vi "FGGA TCP Packet_v3.vi"(7 "TCP Packet In":string, 12 "Data Array":string[](array[string])) -> (8 "TCP Binary Packet":string)   [LabVIEW 2014]
panel:
  out "array":string[](array[string])
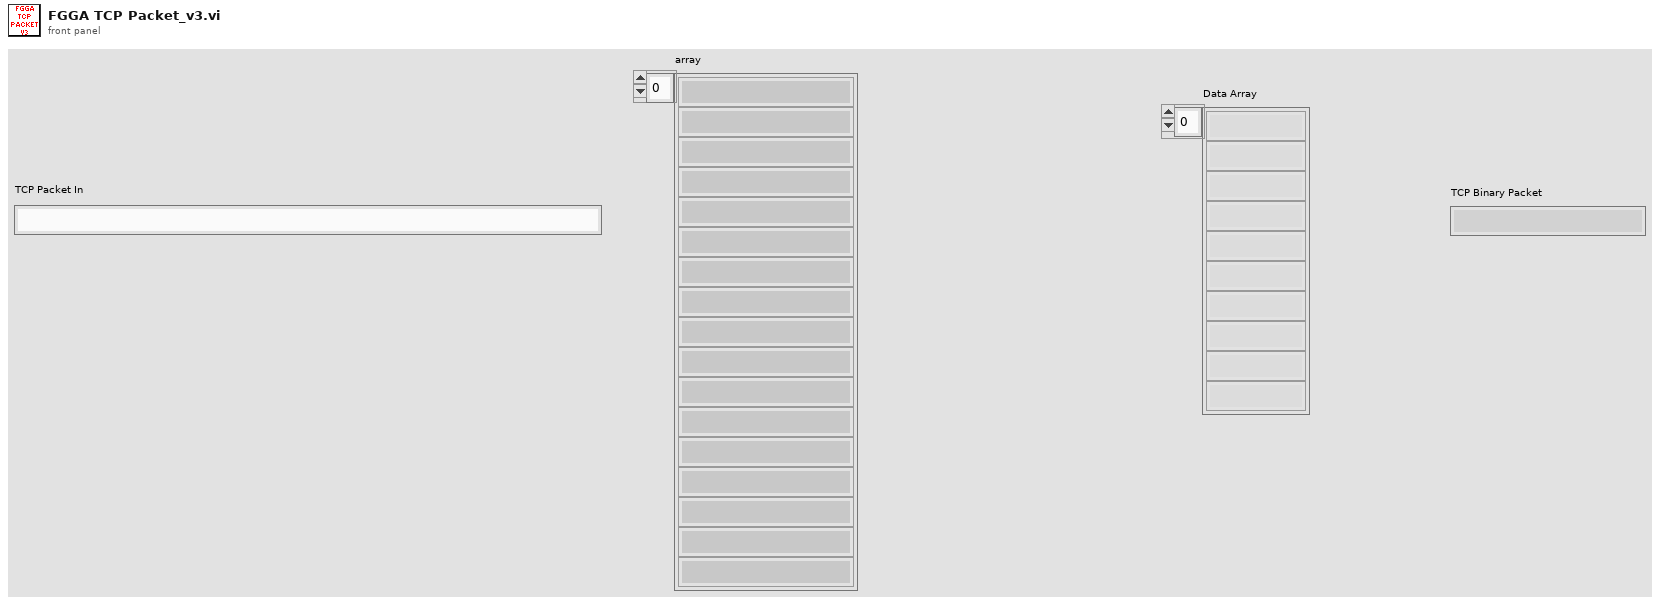
[diagram p1: front panel]
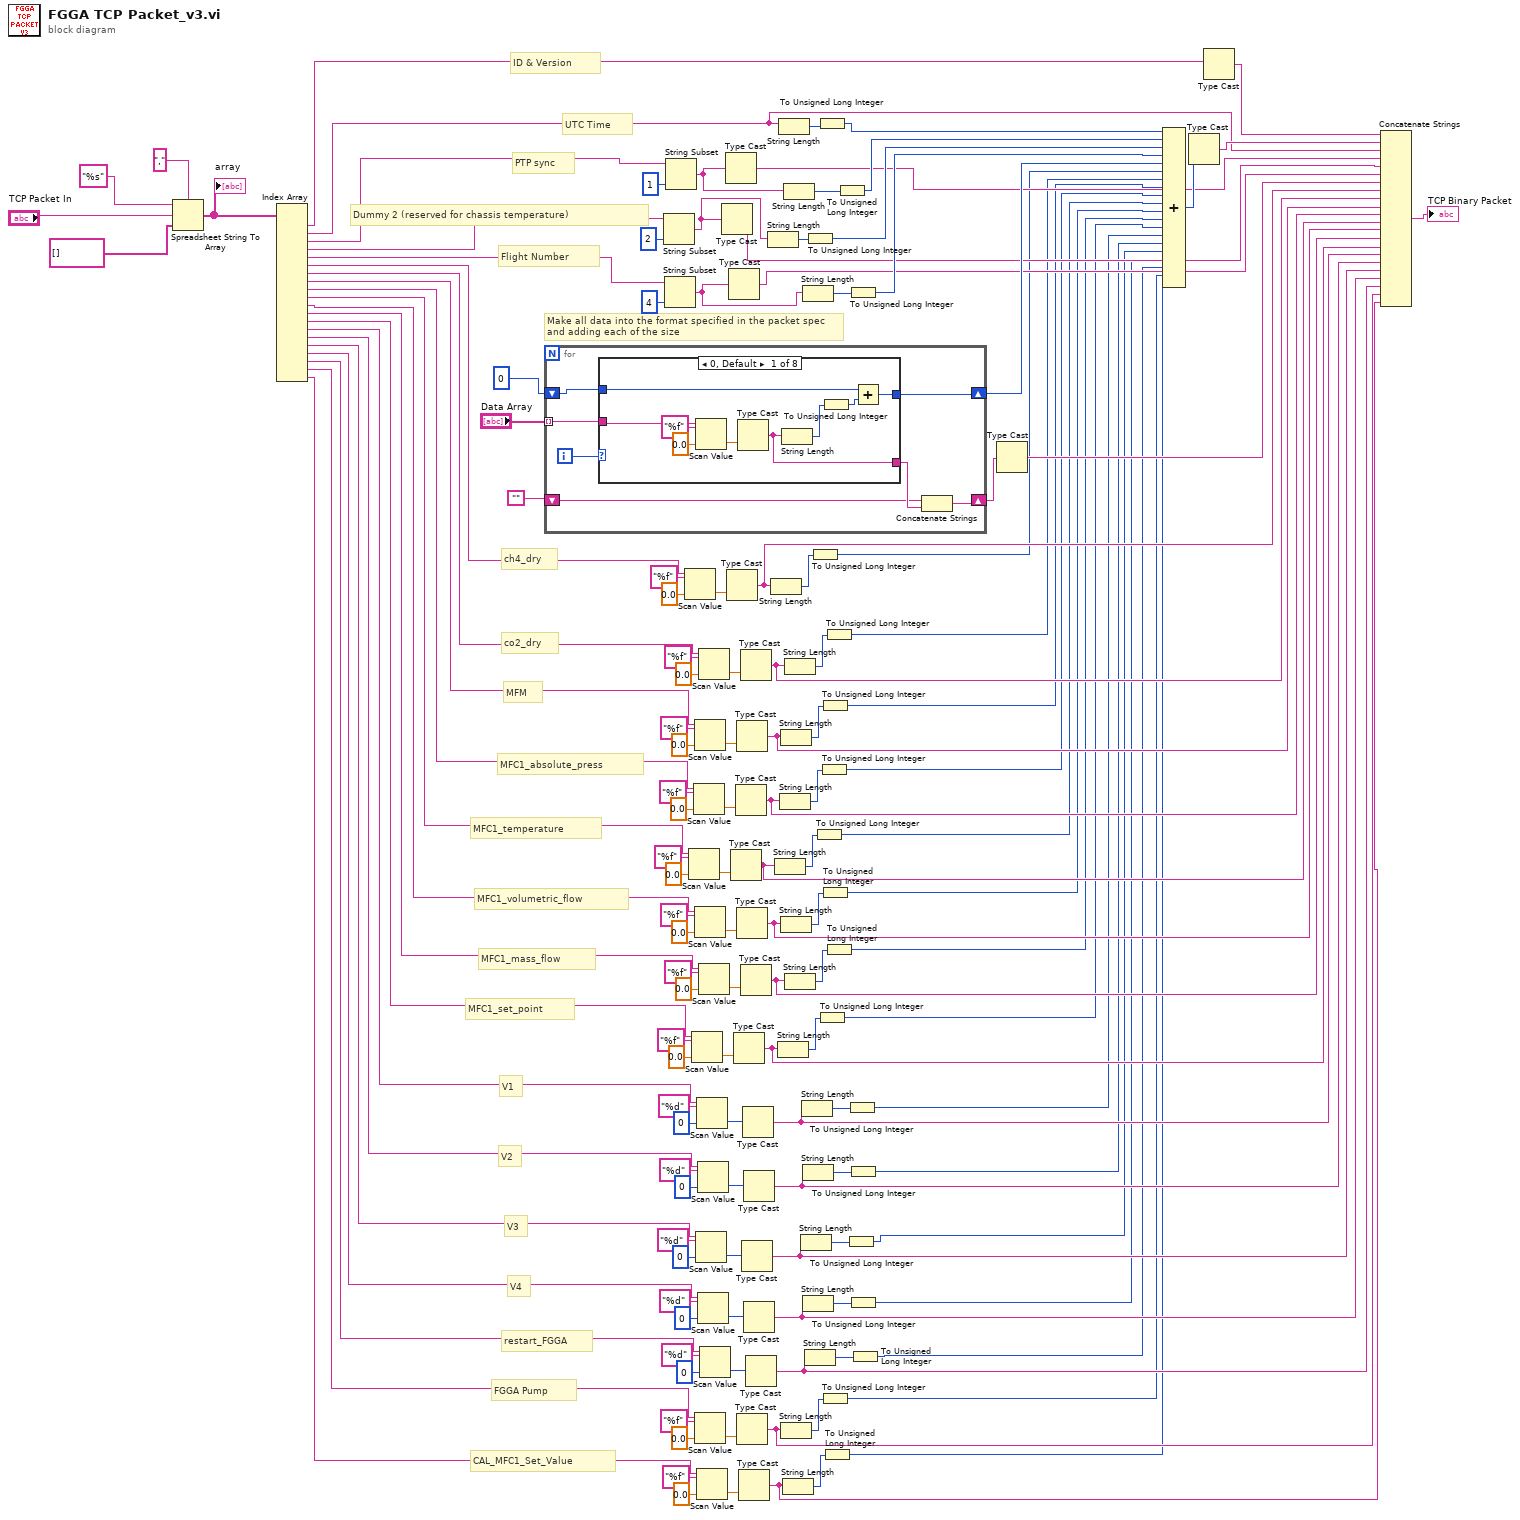
[diagram p0: block diagram]
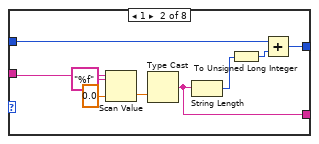
[diagram p2: hidden frame]
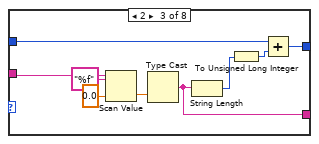
[diagram p3: hidden frame]
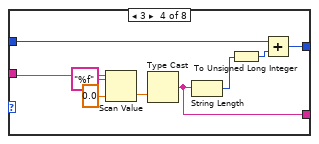
[diagram p4: hidden frame]
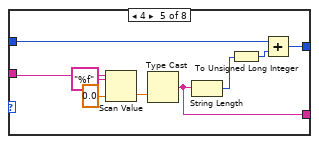
[diagram p5: hidden frame]
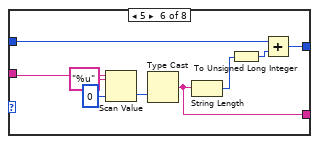
[diagram p6: hidden frame]
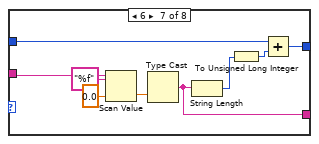
[diagram p7: hidden frame]
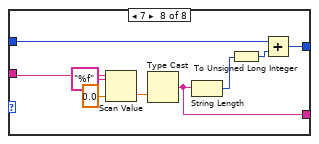
[diagram p8: hidden frame]
diagram:
  # "PTP sync"
  # "CAL_MFC1_Set_Value"
  # "FGGA Pump"
  # "restart_FGGA"
  # "V4"
  # "V3"
  # "V2"
  # "V1"
  # "MFC1_set_point"
  # "MFC1_mass_flow"
  # "MFC1_volumetric_flow"
  # "MFC1_temperature"
  # "MFC1_absolute_press"
  # "MFM"
  # "co2_dry"
  # "ch4_dry"
  # "Flight Number"
  # "Dummy 2 (reserved for chassis temperature)"
  # "UTC Time"
  # "ID & Version"
  # "Make all data into the format specified in the packet spec\nand adding each of the size"
  n1 = Spreadsheet String To Array(delimiter (Tab)=",", format string="%s", spreadsheet string="TCP Packet In", array type (2D Dbl)=string[] []) -> (array=w99:string[])
  "array" <- w99
  n2 = Index Array(array=w99) -> (element #1=w98:string, element #2=w97:string, element #3=w96:string, element #4=w95:string, element #5=w94:string, element #6=w93:string, element #7=w92:string, element #8=w67:string, element #9=w64:string, element #10=w61:string, element #11=w58:string, element #12=w55:string, element #13=w52:string, element #14=w45:string, element #15=w38:string, element #16=w15:string, element #17=w12:string, element #18=w9:string, element #19=w6:string, element #20=w3:string)  [unwired: 20 in]
  n3 = for {
    tunnel: "Data Array" -> [w148] mode=indexing
    shift-right: [w146] -> w130
    shift-left: u32 0 -> [w147]
    shift-right: [w145] -> w119
    shift-left: "" -> [w143]
    i -> [w149]
    n4 = case shown="0, Default" w149 {
      tunnel: w148 -> [w156 w165 w174 w183 w192 w201 w210 w219]
      tunnel: w147 -> [w154 w163 w172 w181 w190 w199 w208 w217]
      tunnel: [w151 w160 w169 w178 w187 w196 w205 w214] -> w146
      tunnel: [w150 w159 w168 w177 w186 w195 w204 w213] -> w144
      frame 0, Default {
        n5 = Scan Value(string=w156, format string="%f", default (0 dbl)=sgl 0.0 ("default (0 I32)")) -> (value=w158:sgl)  [unwired: 1 out]
        n6 = Type Cast(x=w158) -> (*(type *) &x=w150:string)  [unwired: 1 in]
        n7 = String Length(string=w150) -> (length=w153:i32)
        n8 = To Unsigned Long Integer(number=w153) -> (unsigned 32bit integer=w152:u32)
        n9 = Add(x=w154, y=w152) -> (x+y=w151:u32)
      }
      frame 1 {
        n10 = Scan Value(string=w165, format string="%f", default (0 dbl)=sgl 0.0 ("default (0 I32)")) -> (value=w167:sgl)  [unwired: 1 out]
        n11 = Type Cast(x=w167) -> (*(type *) &x=w159:string)  [unwired: 1 in]
        n12 = String Length(string=w159) -> (length=w162:i32)
        n13 = To Unsigned Long Integer(number=w162) -> (unsigned 32bit integer=w161:u32)
        n14 = Add(x=w163, y=w161) -> (x+y=w160:u32)
      }
      frame 2 {
        n15 = Scan Value(string=w174, format string="%f", default (0 dbl)=sgl 0.0 ("default (0 I32)")) -> (value=w176:sgl)  [unwired: 1 out]
        n16 = Type Cast(x=w176) -> (*(type *) &x=w168:string)  [unwired: 1 in]
        n17 = String Length(string=w168) -> (length=w171:i32)
        n18 = To Unsigned Long Integer(number=w171) -> (unsigned 32bit integer=w170:u32)
        n19 = Add(x=w172, y=w170) -> (x+y=w169:u32)
      }
      frame 3 {
        n20 = Scan Value(string=w183, format string="%f", default (0 dbl)=sgl 0.0 ("default (0 I32)")) -> (value=w185:sgl)  [unwired: 1 out]
        n21 = Type Cast(x=w185) -> (*(type *) &x=w177:string)  [unwired: 1 in]
        n22 = String Length(string=w177) -> (length=w180:i32)
        n23 = To Unsigned Long Integer(number=w180) -> (unsigned 32bit integer=w179:u32)
        n24 = Add(x=w181, y=w179) -> (x+y=w178:u32)
      }
      frame 4 {
        n25 = Scan Value(string=w192, format string="%f", default (0 dbl)=sgl 0.0 ("default (0 I32)")) -> (value=w194:sgl)  [unwired: 1 out]
        n26 = Type Cast(x=w194) -> (*(type *) &x=w186:string)  [unwired: 1 in]
        n27 = String Length(string=w186) -> (length=w189:i32)
        n28 = To Unsigned Long Integer(number=w189) -> (unsigned 32bit integer=w188:u32)
        n29 = Add(x=w190, y=w188) -> (x+y=w187:u32)
      }
      frame 5 {
        n30 = Scan Value(string=w201, format string="%u", default (0 dbl)=u16 0 ("default (0 I32)")) -> (value=w203:u16)  [unwired: 1 out]
        n31 = Type Cast(x=w203) -> (*(type *) &x=w195:string)  [unwired: 1 in]
        n32 = String Length(string=w195) -> (length=w198:i32)
        n33 = To Unsigned Long Integer(number=w198) -> (unsigned 32bit integer=w197:u32)
        n34 = Add(x=w199, y=w197) -> (x+y=w196:u32)
      }
      frame 6 {
        n35 = Scan Value(string=w210, format string="%f", default (0 dbl)=sgl 0.0 ("default (0 I32)")) -> (value=w212:sgl)  [unwired: 1 out]
        n36 = Type Cast(x=w212) -> (*(type *) &x=w204:string)  [unwired: 1 in]
        n37 = String Length(string=w204) -> (length=w207:i32)
        n38 = To Unsigned Long Integer(number=w207) -> (unsigned 32bit integer=w206:u32)
        n39 = Add(x=w208, y=w206) -> (x+y=w205:u32)
      }
      frame 7 {
        n40 = Scan Value(string=w219, format string="%f", default (0 dbl)=sgl 0.0 ("default (0 I32)")) -> (value=w221:sgl)  [unwired: 1 out]
        n41 = Type Cast(x=w221) -> (*(type *) &x=w213:string)  [unwired: 1 in]
        n42 = String Length(string=w213) -> (length=w216:i32)
        n43 = To Unsigned Long Integer(number=w216) -> (unsigned 32bit integer=w215:u32)
        n44 = Add(x=w217, y=w215) -> (x+y=w214:u32)
      }
    }
    n45 = Concatenate Strings(w143, w144) -> (w145:string)
  }
  n46 = String Subset(string=w95, length (rest)=2 ("length (rest)")) -> (substring=w117:string)  [unwired: 1 in]
  n47 = String Subset(string=w94, length (rest)=4 ("length (rest)")) -> (substring=w123:string)  [unwired: 1 in]
  n48 = String Subset(string=w96, length (rest)=1 ("length (rest)")) -> (substring=w126:string)  [unwired: 1 in]
  n49 = Scan Value(string=w93, format string="%f", default (0 dbl)=sgl 0.0 ("default (0 I32)")) -> (value=w115:sgl)  [unwired: 1 out]
  n50 = Scan Value(string=w61, format string="%f", default (0 dbl)=sgl 0.0 ("default (0 I32)")) -> (value=w83:sgl)  [unwired: 1 out]
  n51 = Scan Value(string=w52, format string="%f", default (0 dbl)=sgl 0.0 ("default (0 I32)")) -> (value=w71:sgl)  [unwired: 1 out]
  n52 = Scan Value(string=w64, format string="%f", default (0 dbl)=sgl 0.0 ("default (0 I32)")) -> (value=w87:sgl)  [unwired: 1 out]
  n53 = Scan Value(string=w67, format string="%f", default (0 dbl)=sgl 0.0 ("default (0 I32)")) -> (value=w91:sgl)  [unwired: 1 out]
  n54 = Scan Value(string=w58, format string="%f", default (0 dbl)=sgl 0.0 ("default (0 I32)")) -> (value=w79:sgl)  [unwired: 1 out]
  n55 = Scan Value(string=w6, format string="%f", default (0 dbl)=sgl 0.0 ("default (0 I32)")) -> (value=w23:sgl)  [unwired: 1 out]
  n56 = Scan Value(string=w15, format string="%d", default (0 dbl)=u16 0 ("default (0 I32)")) -> (value=w32:u16)  [unwired: 1 out]
  n57 = Scan Value(string=w45, format string="%d", default (0 dbl)=u16 0 ("default (0 I32)")) -> (value=w46:u16)  [unwired: 1 out]
  n58 = Scan Value(string=w3, format string="%f", default (0 dbl)=sgl 0.0 ("default (0 I32)")) -> (value=w19:sgl)  [unwired: 1 out]
  n59 = Scan Value(string=w38, format string="%d", default (0 dbl)=u16 0 ("default (0 I32)")) -> (value=w39:u16)  [unwired: 1 out]
  n60 = Scan Value(string=w12, format string="%d", default (0 dbl)=u16 0 ("default (0 I32)")) -> (value=w28:u16)  [unwired: 1 out]
  n61 = Scan Value(string=w92, format string="%f", default (0 dbl)=sgl 0.0 ("default (0 I32)")) -> (value=w109:sgl)  [unwired: 1 out]
  n62 = Scan Value(string=w55, format string="%f", default (0 dbl)=sgl 0.0 ("default (0 I32)")) -> (value=w75:sgl)  [unwired: 1 out]
  n63 = Scan Value(string=w9, format string="%d", default (0 dbl)=u16 0 ("default (0 I32)")) -> (value=w24:u16)  [unwired: 1 out]
  n64 = Type Cast(x=w117) -> (*(type *) &x=w116:string)  [unwired: 1 in]
  n65 = Type Cast(x=w126) -> (*(type *) &x=w125:string)  [unwired: 1 in]
  n66 = Type Cast(x=w115) -> (*(type *) &x=w111:string)  [unwired: 1 in]
  n67 = Type Cast(x=w123) -> (*(type *) &x=w124:string)  [unwired: 1 in]
  n68 = Type Cast(x=w83) -> (*(type *) &x=w59:string)  [unwired: 1 in]
  n69 = Type Cast(x=w71) -> (*(type *) &x=w50:string)  [unwired: 1 in]
  n70 = Type Cast(x=w87) -> (*(type *) &x=w62:string)  [unwired: 1 in]
  n71 = Type Cast(x=w91) -> (*(type *) &x=w65:string)  [unwired: 1 in]
  n72 = Type Cast(x=w79) -> (*(type *) &x=w56:string)  [unwired: 1 in]
  n73 = Type Cast(x=w23) -> (*(type *) &x=w4:string)  [unwired: 1 in]
  n74 = Type Cast(x=w19) -> (*(type *) &x=w1:string)  [unwired: 1 in]
  n75 = Type Cast(x=w109) -> (*(type *) &x=w104:string)  [unwired: 1 in]
  n76 = Type Cast(x=w75) -> (*(type *) &x=w53:string)  [unwired: 1 in]
  n77 = Type Cast(x=w32) -> (*(type *) &x=w13:string)  [unwired: 1 in]
  n78 = Type Cast(x=w46) -> (*(type *) &x=w43:string)  [unwired: 1 in]
  n79 = Type Cast(x=w39) -> (*(type *) &x=w36:string)  [unwired: 1 in]
  n80 = Type Cast(x=w28) -> (*(type *) &x=w10:string)  [unwired: 1 in]
  n81 = Type Cast(x=w24) -> (*(type *) &x=w7:string)  [unwired: 1 in]
  n82 = String Length(string=w117) -> (length=w137:i32)
  n83 = String Length(string=w111) -> (length=w112:i32)
  n84 = String Length(string=w59) -> (length=w80:i32)
  n85 = String Length(string=w50) -> (length=w68:i32)
  n86 = String Length(string=w97) -> (length=w142:i32)
  n87 = String Length(string=w62) -> (length=w84:i32)
  n88 = String Length(string=w65) -> (length=w88:i32)
  n89 = String Length(string=w56) -> (length=w76:i32)
  n90 = String Length(string=w4) -> (length=w20:i32)
  n91 = String Length(string=w1) -> (length=w16:i32)
  n92 = String Length(string=w126) -> (length=w139:i32)
  n93 = String Length(string=w104) -> (length=w106:i32)
  n94 = String Length(string=w53) -> (length=w72:i32)
  n95 = String Length(string=w13) -> (length=w35:i32)
  n96 = String Length(string=w43) -> (length=w49:i32)
  n97 = String Length(string=w123) -> (length=w134:i32)
  n98 = String Length(string=w36) -> (length=w42:i32)
  n99 = String Length(string=w10) -> (length=w31:i32)
  n100 = To Unsigned Long Integer(number=w137) -> (unsigned 32bit integer=w136:u32)
  n101 = String Length(string=w7) -> (length=w27:i32)
  n102 = To Unsigned Long Integer(number=w112) -> (unsigned 32bit integer=w110:u32)
  n103 = To Unsigned Long Integer(number=w80) -> (unsigned 32bit integer=w60:u32)
  n104 = To Unsigned Long Integer(number=w142) -> (unsigned 32bit integer=w141:u32)
  n105 = To Unsigned Long Integer(number=w68) -> (unsigned 32bit integer=w51:u32)
  n106 = To Unsigned Long Integer(number=w84) -> (unsigned 32bit integer=w63:u32)
  n107 = To Unsigned Long Integer(number=w88) -> (unsigned 32bit integer=w66:u32)
  n108 = To Unsigned Long Integer(number=w76) -> (unsigned 32bit integer=w57:u32)
  n109 = To Unsigned Long Integer(number=w20) -> (unsigned 32bit integer=w5:u32)
  n110 = To Unsigned Long Integer(number=w16) -> (unsigned 32bit integer=w2:u32)
  n111 = To Unsigned Long Integer(number=w106) -> (unsigned 32bit integer=w105:u32)
  n112 = To Unsigned Long Integer(number=w72) -> (unsigned 32bit integer=w54:u32)
  n113 = To Unsigned Long Integer(number=w139) -> (unsigned 32bit integer=w138:u32)
  n114 = To Unsigned Long Integer(number=w35) -> (unsigned 32bit integer=w14:u32)
  n115 = To Unsigned Long Integer(number=w49) -> (unsigned 32bit integer=w44:u32)
  n116 = To Unsigned Long Integer(number=w134) -> (unsigned 32bit integer=w133:u32)
  n117 = To Unsigned Long Integer(number=w42) -> (unsigned 32bit integer=w37:u32)
  n118 = To Unsigned Long Integer(number=w31) -> (unsigned 32bit integer=w11:u32)
  n119 = To Unsigned Long Integer(number=w27) -> (unsigned 32bit integer=w8:u32)
  n120 = Type Cast(x=w119) -> (*(type *) &x=w122:string)  [unwired: 1 in]
  n121 = Compound Arithmetic op=ADD(w141, w138, w136, w133, w130, w110, w105, w66, w63, w60, w57, w54, w51, w44, w37, w14, w11, w8, w5, w2) -> (w128:u32)
  n122 = Type Cast(x=w128) -> (*(type *) &x=w127:string)  [unwired: 1 in]
  n123 = Type Cast(x=w98) -> (*(type *) &x=w129:string)  [unwired: 1 in]
  n124 = Concatenate Strings(w129, w127, w97, w125, w116, w124, w122, w111, w104, w65, w62, w59, w56, w53, w50, w43, w36, w13, w10, w7, w4, w1) -> (→"TCP Binary Packet":string)
